vi "Type.Convert.String.vi"(10 "Direction":T1(ring), 11 "Type":T2) -> (2 "ArbIDName":string, 3 "Service Name":string)   [LabVIEW 2024, in "Diagnostics Addon Engine.lvlib"]
uses:
  Diagnostics Addon Engine.lvlib
  Addon Shared/Types/Type.ctl
  Addon Shared/Diagnostics Addon Shared.lvlib
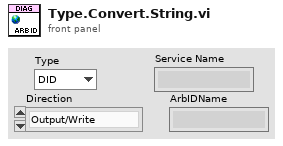
[diagram p1: front panel]
types:
  T1 = enum16{"Output/Write", "Input/Read", "Input/ReadWrite"}
  T2 = typedef "Diagnostics Addon Shared.lvlib/Type.ctl" = enum16{"DID", "CDID", "PID", "CPID", "Read Memory", "Write Memory", "IO Control", "Routine Start", "Routine Request", "Routine Stop", "User Defined", "DTC Control", "Clear DTCs", "Read DTCs", "Start DTCs", "DTC Change Count", "Tester Present", "Unlock ECU", "Reset ECU", "Diag Session Control", "Communication Control", "DPID Control", "Poll Control", "Diag Comm Port Control"}
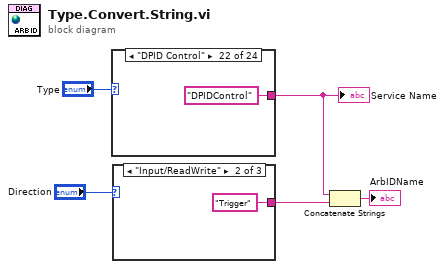
[diagram p0: block diagram]
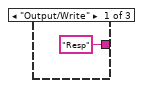
[diagram p2: hidden frame]
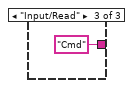
[diagram p3: hidden frame]
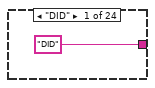
[diagram p4: hidden frame]
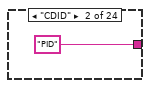
[diagram p5: hidden frame]
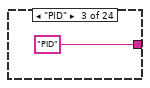
[diagram p6: hidden frame]
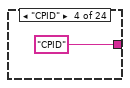
[diagram p7: hidden frame]
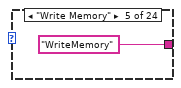
[diagram p8: hidden frame]
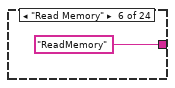
[diagram p9: hidden frame]
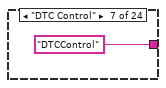
[diagram p10: hidden frame]
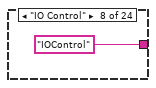
[diagram p11: hidden frame]
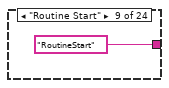
[diagram p12: hidden frame]
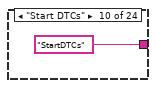
[diagram p13: hidden frame]
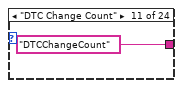
[diagram p14: hidden frame]
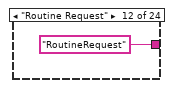
[diagram p15: hidden frame]
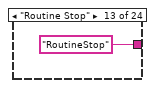
[diagram p16: hidden frame]
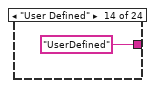
[diagram p17: hidden frame]
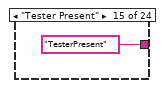
[diagram p18: hidden frame]
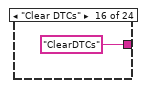
[diagram p19: hidden frame]
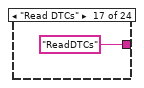
[diagram p20: hidden frame]
diagram:
  n1 = case shown="\"DPID Control\"" "Type" {
    tunnel: ["DID" ("signal name") "PID" ("signal name") "PID" ("signal name") "CPID" ("signal name") "WriteMemory" ("signal name") "ReadMemory" ("signal name") "DTCControl" ("signal name") "IOControl" ("signal name") "RoutineStart" ("signal name") "StartDTCs" ("signal name") "DTCChangeCount" ("signal name") "RoutineRequest" ("signal name") "RoutineStop" ("signal name") "UserDefined" ("signal name") "TesterPresent" ("signal name") "ClearDTCs" ("signal name") "ReadDTCs" ("signal name") "UnlockECU" ("signal name") "ResetECU" ("signal name") "DiagSessionControl" ("signal name") "NormComm" ("signal name") "DPIDControl" ("signal name") "PollControl" ("signal name") "DiagCANControl" ("signal name")] -> w2
    frame "DID" {
    }
    frame "CDID" {
    }
    frame "PID" {
    }
    frame "CPID" {
    }
    frame "Write Memory" {
    }
    frame "Read Memory" {
    }
    frame "DTC Control" {
    }
    frame "IO Control" {
    }
    frame "Routine Start" {
    }
    frame "Start DTCs" {
    }
    frame "DTC Change Count" {
    }
    frame "Routine Request" {
    }
    frame "Routine Stop" {
    }
    frame "User Defined" {
    }
    frame "Tester Present" {
    }
    frame "Clear DTCs" {
    }
    frame "Read DTCs" {
    }
    frame "Unlock ECU" {
    }
    frame "Reset ECU" {
    }
    frame "Diag Session Control" {
    }
    frame "Communication Control" {
    }
    frame "DPID Control" {
    }
    frame "Poll Control" {
    }
    frame "Diag Comm Port Control" {
    }
  }
  "Service Name" <- w2
  n2 = case shown="\"Input/ReadWrite\"" "Direction" {
    tunnel: ["Resp" ("signal name") "Trigger" ("signal name") "Cmd" ("signal name")] -> w3
    frame "Output/Write" {
    }
    frame "Input/ReadWrite" {
    }
    frame "Input/Read" {
    }
  }
  n3 = Concatenate Strings(w2, w3) -> (→"ArbIDName":string)
